vi "Parse All Package Names.vi"(11 "index.vipr":string) -> (3 "All Packages":T1[](array[typedef]))   [LabVIEW 2016, in "Packages.lvlib" / "VIPM.lvlib"]
uses:
  VIPM.lvlib
  Package--cluster.ctl
  Packages.lvlib
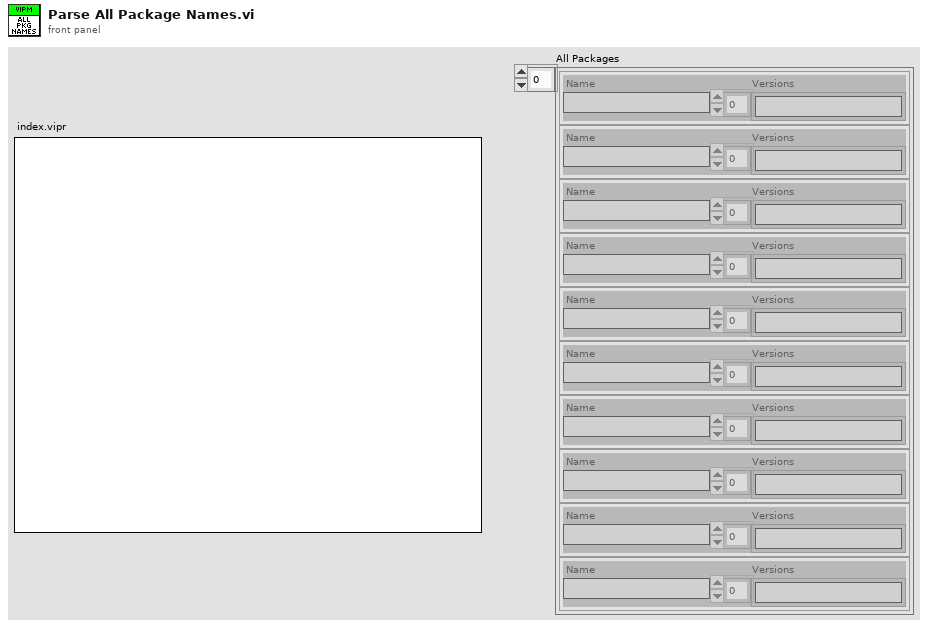
[diagram p1: front panel]
types:
  T1 = typedef "Packages.lvlib/Package--cluster.ctl" = cluster{"Name":string, "Versions":string[]}
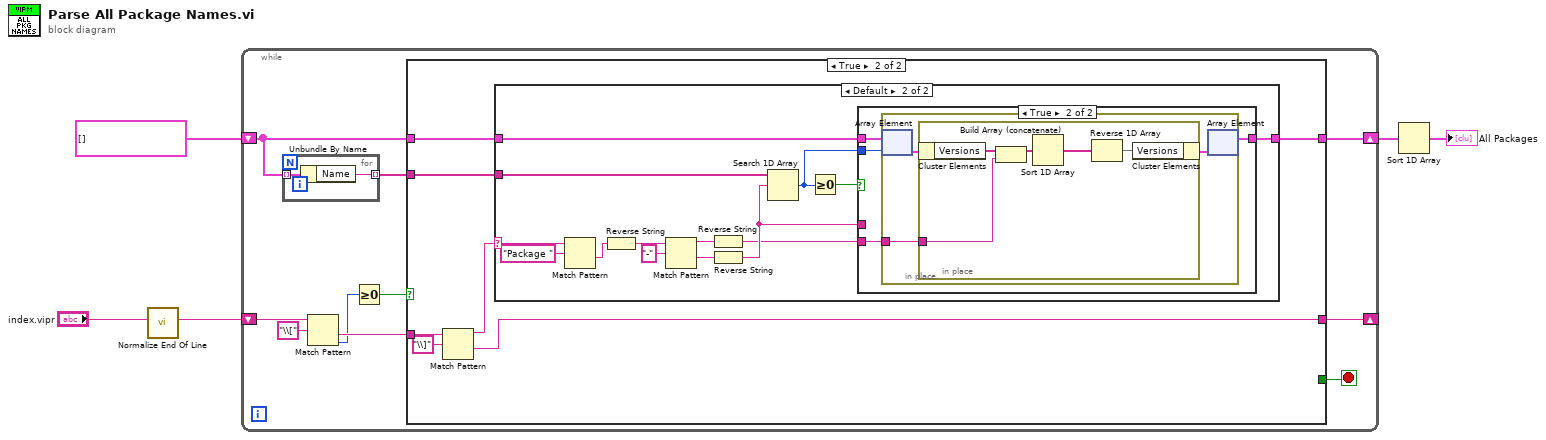
[diagram p0: block diagram]
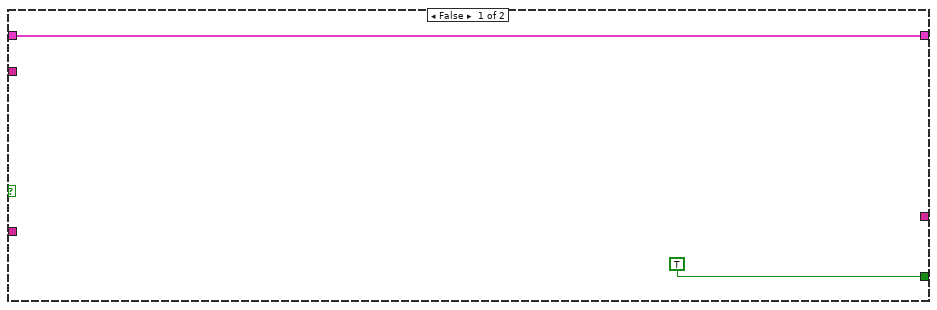
[diagram p2: hidden frame]
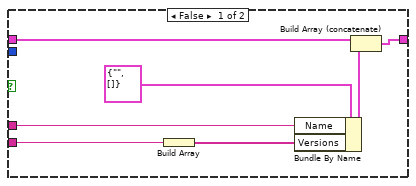
[diagram p4: hidden frame]
diagram:
  n1 = call <vilib>:"Normalize End Of Line.vi"("string in"="index.vipr") -> ("string out"=w2:string)  [unwired: 7 in]
  n2 = while {
    shift-right: [w12] -> _
    shift-left: w2 -> [w15]
    shift-right: [w9] -> w3
    shift-left: T1[] [] -> [w8]
    stop <- w6 stop-if-true
    n3 = for {
      tunnel: w8 -> [w60] mode=indexing
      tunnel: [w59] -> w10 mode=indexing
      n4 = Unbundle By Name(w60) -> ("Name"=w59:string)
    }
    n5 = Match Pattern(string=w15, regular expression="\\[") -> (after substring=w13:string, offset past match=w11:i32)  [unwired: 1 in, 2 out]
    n6 = Greater Or Equal To 0?(x=w11) -> (x >= 0?=w7:bool)
    n7 = case shown="True" w7 {
      tunnel: w13 -> [_ w24]
      tunnel: [_ w22] -> w12
      tunnel: w10 -> [_ w21]
      tunnel: [w17 w20] -> w9
      tunnel: w8 -> [w17 w19]
      tunnel: [TRUE _] -> w6
      frame False {
      }
      frame True {
        n8 = Match Pattern(string=w24, regular expression="\\]") -> (before substring=w18:string, after substring=w22:string)  [unwired: 1 in, 2 out]
        n9 = case shown="Default" w18 {
          selector: w18 -> [_ w29]
          tunnel: w21 -> [_ w35]
          tunnel: [w25 w33] -> w20
          tunnel: w19 -> [w25 w32]
          frame "Self" {
          }
          frame Default {
            n10 = Match Pattern(string=w29, regular expression="Package ") -> (after substring=w28:string)  [unwired: 1 in, 3 out]
            n11 = Reverse String(1:w28) -> (0:w39:string)
            n12 = Match Pattern(string=w39, regular expression="-") -> (before substring=w37:string, after substring=w36:string)  [unwired: 1 in, 2 out]
            n13 = Reverse String(1:w37) -> (0:w26:string)
            n14 = Reverse String(1:w36) -> (0:w31:string)
            n15 = Search 1D Array(1D array=w35, element=w31) -> (index of element=w30:i32)  [unwired: 1 in]
            n16 = Greater Or Equal To 0?(x=w30) -> (x >= 0?=w34:bool)
            n17 = case shown="True" w34 {
              tunnel: [w45 w48] -> w33
              tunnel: w32 -> [w46 w50]
              tunnel: w31 -> [w42 _]
              tunnel: w26 -> [w41 w47]
              tunnel: w30 -> [_ w49]
              frame False {
                n18 = Build Array(w41) -> (w40:string[])
                n19 = Bundle By Name(cluster=T1 {"Name"="", "Versions"=[]} ("array"), "Name"=w42, "Versions"=w40) -> (w43:T1)
                n20 = Build Array (concatenate)(w46, w43) -> (w45:T1[])
              }
              frame True {
                n21 = in-place {
                  in-place-border: w47 -> [w51]
                  n22 = in-place-array #1(w50, w49) -> (w53:T1)
                  n23 = in-place {
                    in-place-border: w51 -> [w56]
                    n24 = in-place-cluster #2(w53) -> ("Versions"=w58:string[])
                    n25 = Build Array (concatenate)(w58, w56) -> (w57:string[])
                    n26 = Sort 1D Array(array=w57) -> (sorted array=w55:string[])
                    n27 = Reverse 1D Array(array=w55) -> (reversed array=w54:string[])
                    n28 = in-place-cluster #2("Versions"=w54) -> (w52:T1)
                  }
                  n29 = in-place-array #1(w52) -> (w48:T1[])  [unwired: 1 out]
                }
              }
            }
          }
        }
      }
    }
  }
  n30 = Sort 1D Array(array=w3) -> (sorted array=→"All Packages":T1[])
